vi "Step Move Z.vi"(2 "Error In":errorcluster, 3 "Direction":bool=TRUE, 4 "No. of Z Steps":string="0", 5 "Reference In":refnum<class "_Controller.lvclass">) -> (0 "Error Out":errorcluster, 1 "Reference Out":refnum<class "_Controller.lvclass">)   [LabVIEW 2020]
doc: "Moves the XYZ scanning machine in the Z-direction. \n\nArgs:\n\nReference In: Incoming communication (reference) between LabView and the scanning rig controller\nError In: Checks for any errors with the incoming communication (reference)\nNo. of Z Steps: Number of steps the motor needs to move\nDirection: Boolean to control the direction the motor moves in \n\nReturns: \n\nReference Out: Output communnication (reference) between LabView and controller\nError Out: Checks for any error with output communication (reference)"
uses:
  <instrlib>/Arcus Ethernet Driver 1.0.0/ArcusEthernetComm/classes/Controller/_Controller.lvclass
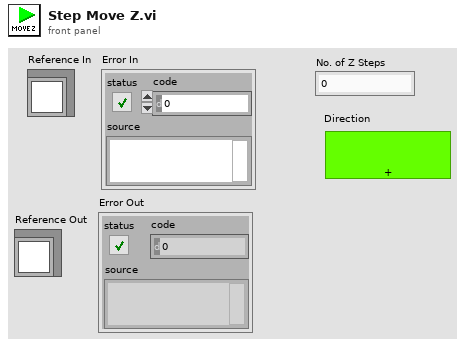
[diagram p1: front panel]
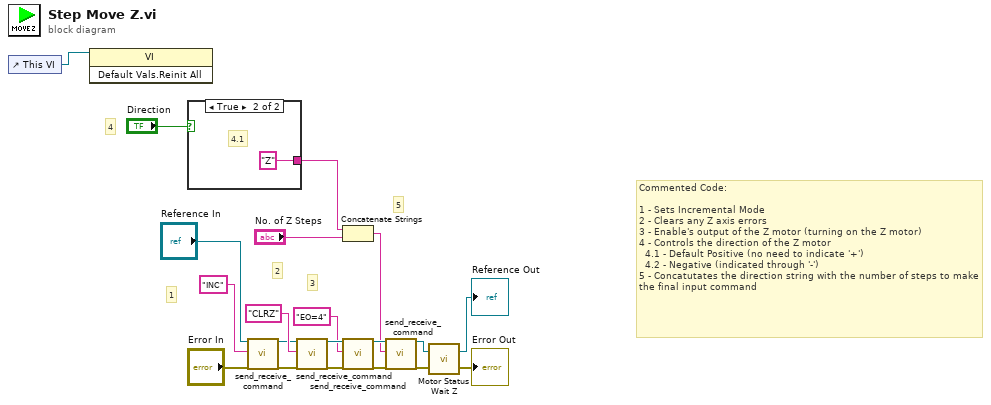
[diagram p0: block diagram]
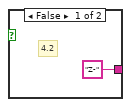
[diagram p2: hidden frame]
diagram:
  # "5"
  # "4"
  # "3"
  # "2"
  # "1"
  # "Commented Code:\n\n1 - Sets Incremental Mode \n2 - Clears any Z axis errors\n3 - Enable's output of the Z motor (turning on the Z motor)\n4 - Controls the direction of the Z motor\n  4.1 - Default Positive (no need to indicate '+')\n  4.2 - Negative (indicated through '-') \n5 - Concatutates the direction string with the number of steps to make the final input command"
  n1 = control-ref of="This VI"() -> (w1:refnum<vi>)
  n2 = invoke class="VI" method="Default Vals.Reinit All"(reference=w1) -> ()  [unwired: 2 in, 3 out]
  n3 = case shown="True" "Direction" {
    tunnel: ["Z-" ("string") "Z" ("string")] -> w6
    frame False {
      # "4.2"
    }
    frame True {
      # "4.1"
    }
  }
  n4 = call <instrlib>:"send_receive_command.vi"("reference (in)"="Reference In", "ASCII Command (in)"="INC", "error in (no error)"="Error In") -> ("reference (out)"=w11:refnum<class "_Controller.lvclass">, "error out"=w8:errorcluster)  [unwired: 12 in, 3 out]
  n5 = call <instrlib>:"send_receive_command.vi"("reference (in)"=w11, "ASCII Command (in)"="CLRZ", "error in (no error)"=w8) -> ("reference (out)"=w18:refnum<class "_Controller.lvclass">, "error out"=w19:errorcluster)  [unwired: 12 in, 3 out]
  n6 = Concatenate Strings(w6, "No. of Z Steps") -> (w14:string)
  n7 = call <instrlib>:"send_receive_command.vi"("reference (in)"=w18, "ASCII Command (in)"="EO=4", "error in (no error)"=w19) -> ("reference (out)"=w16:refnum<class "_Controller.lvclass">, "error out"=w17:errorcluster)  [unwired: 12 in, 3 out]
  n8 = call <instrlib>:"send_receive_command.vi"("reference (in)"=w16, "ASCII Command (in)"=w14, "error in (no error)"=w17) -> ("reference (out)"=w5:refnum<class "_Controller.lvclass">, "error out"=w4:errorcluster)  [unwired: 12 in, 3 out]
  n9 = call "Motor Status Wait Z.vi"("Error In"=w4, "Reference In"=w5) -> ("Error Out"=→"Error Out":errorcluster, "Reference Out"=→"Reference Out":refnum<class "_Controller.lvclass">)
